vi "SPCInitializeTrigger.vi"(1 "timing info":cluster{"Fs":dbl, "#s":dbl} {"#s" format="%.2f"; "Fs" format="%.2f"}, 2 "Image Settings":T1={"Start Position (µm)"={"x"=0.0, "y"=0.0, "z"=0.0}, "End Position (µm)"={"x"=10.0, "y"=10.0, "z"=0.0}, "Image Resolution (nm/pixel)"={"x"=50.0, "y"=50.0, "z"=100.0}, "Image Size (µm)"={"x"=10.0, "y"=10.0, "z"=0.0}, "Image Size (pixel)"={"x"=50, "y"=50, "z"=0}, "Time Resolution\n(ms/pixel)"=7.0, "1st Axis"=0, "2nd Axis"=1, "Retrace"=FALSE, "Estimated Time"=""} {"2nd Axis" items=["x", "y", "z"]; "1st Axis" items=["x", "y", "z"]; "Time Resolution\n(ms/pixel)" format="%.2f"; "Image Resolution (nm/pixel)"."z" format="%.2f"; "Image Resolution (nm/pixel)"."y" format="%.2f"; "Image Resolution (nm/pixel)"."x" format="%.2f"; "Image Size (µm)"."z" format="%.2f"; "Image Size (µm)"."y" format="%.2f"; "Image Size (µm)"."x" format="%.2f"; "End Position (µm)"."z" format="%.2f"; "End Position (µm)"."y" format="%.2f"; "End Position (µm)"."x" format="%.2f"; "Start Position (µm)"."z" format="%.2f"; "Start Position (µm)"."y" format="%.2f"; "Start Position (µm)"."x" format="%.2f"}) -> (0 "signal out":T2)   [LabVIEW 2009]
uses:
  AnalogTrace.ctt
  ImageSettings.ctt
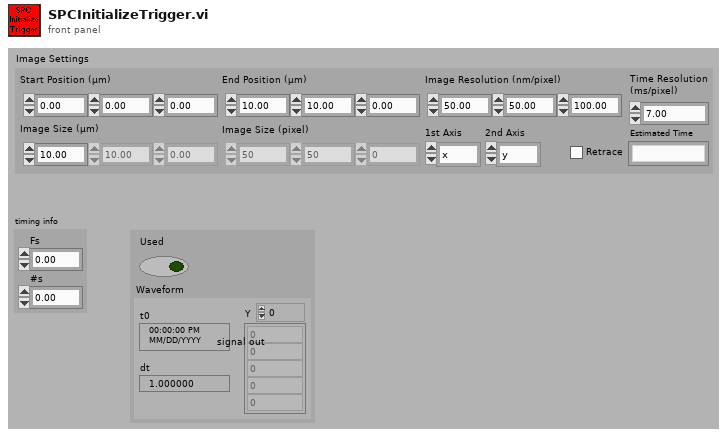
[diagram p1: front panel]
types:
  T1 = typedef "ImageSettings.ctt" = cluster{"Start Position (µm)":cluster{"x":dbl, "y":dbl, "z":dbl}, "End Position (µm)":cluster{"x":dbl, "y":dbl, "z":dbl}, "Image Resolution (nm/pixel)":cluster{"x":dbl, "y":dbl, "z":dbl}, "Image Size (µm)":cluster{"x":dbl, "y":dbl, "z":dbl}, "Image Size (pixel)":cluster{"x":u32, "y":u32, "z":u32}, "Time Resolution\n(ms/pixel)":dbl, "1st Axis":u16, "2nd Axis":u16, "Retrace":bool, "Estimated Time":string}
  T2 = typedef "AnalogTrace.ctt" = cluster{"Used":bool, "Waveform":waveform(dbl)}
  T3 = typedef "FIFOSettings.ctt" = cluster{"Measurement":cluster{"Binning (ms)":sgl, "External Trigger Condition":u16, "Stop Condition:":u16, "Stop Count":dbl, "Buffer Size (Photons)":u32, "No of Channels":u16, "Ext Latch Delay":i16}, "ADC":cluster{"Binning (HH)":i16, "Dither Range":i16, "Count Increment":i16, "Mode":u16}, "SYNC":cluster{"SYNC ZC Level (mV)":sgl, "SYNC Freq Divider":u16, "SYNC Holdoff (ps)":sgl, "SYNC Threshold (mV)":sgl}, "TAC":cluster{"TAC Range (ns)":sgl, "TAC Gain":i16, "TAC Offset (%)":sgl, "TAC Limit Low (%)":sgl, "TAC Limit High (%)":sgl}, "Ch 2":cluster{"Ch2 ZC Level (mV)":sgl, "Ch2 Holdoff (ps)":sgl, "Ch2 Threshold (mV)":sgl}, "Ch 3":cluster{"Ch3 ZC Level (mV)":sgl, "Ch3 Holdoff (ps)":sgl, "Ch3 Threshold (mV)":sgl}, "Ch 4":cluster{"Ch4 ZC Level (mV)":sgl, "Ch4 Holdoff (ps)":sgl, "Ch4 Threshold (mV)":sgl}, "Ch1":cluster{"Ch1 ZC Level (mV)":sgl, "Ch1 Holdoff (ps)":sgl, "Ch1 Threshold (mV)":sgl}}
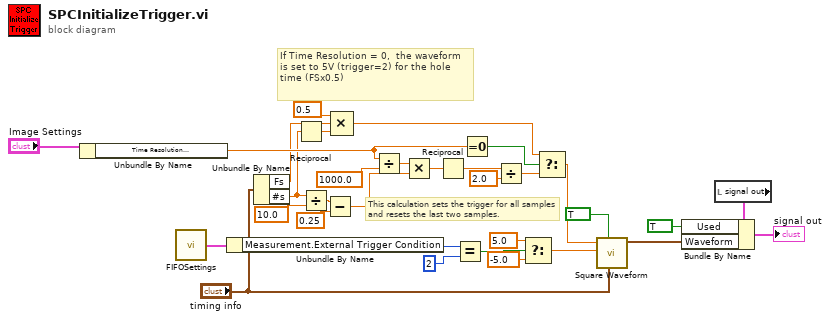
[diagram p0: block diagram]
diagram:
  # "If Time Resolution = 0,  the waveform is set to 5V (trigger=2) for the hole time (FSx0.5)"
  # "This calculation sets the trigger for all samples\nand resets the last two samples."
  n1 = Unbundle By Name("Image Settings") -> ("Time Resolution\n(ms/pixel)"=w6:dbl)
  n2 = call "FIFOSettings.vi"() -> ("FIFO Settings(out)"=w32:T3)  [unwired: 2 in]
  n3 = Unbundle By Name(w32) -> ("Measurement.External Trigger Condition"=w31:u16)
  n4 = Unbundle By Name("timing info") -> ("Fs"=w5:dbl, "#s"=w2:dbl)
  n5 = Reciprocal(x=w2) -> (1/x=w3:dbl)
  n6 = Divide(x=w2, y=10.0) -> (x/y=w16:dbl)
  n7 = Subtract(x=w16, y=0.25) -> (x-y=w13:dbl)
  n8 = Compound Arithmetic op=MULTIPLY(0.5 ("value"), w5, w3) -> (w4:dbl)
  n9 = Divide(x=w6, y=1000.0) -> (x/y=w14:dbl)
  n10 = Multiply(x=w14, y=w13) -> (x*y=w12:dbl)
  n11 = Reciprocal(x=w12) -> (1/x=w18:dbl)
  n12 = Equal?(x=w31, y=u16 2) -> (x = y?=w27:bool)
  n13 = Equal To 0?(x=w6) -> (x = 0?=w7:bool)
  n14 = Divide(x=w18, y=2.0) -> (x/y=w8:dbl)
  n15 = Select(t=5.0, s=w27, f=-5.0) -> (s? t:f=w21:dbl)
  n16 = Select(t=w4, s=w7, f=w8) -> (s? t:f=w9:dbl)
  n17 = call "Square Waveform.vi"("sampling info"="timing info", "reset signal"=TRUE, "amplitude"=w21, "frequency"=w9) -> ("signal out"=w22:waveform(dbl))  [unwired: 6 in, 1 out]
  n18 = local read "signal out"() -> (w26:T2)
  n19 = Bundle By Name(cluster=w26, "Used"=TRUE, "Waveform"=w22) -> (→"signal out":T2)
